vi "Config ACTION.vi"(8 "error in (no error)":errorcluster, 11 "Measurement in":refnum<class "Measurement.lvclass">) -> (0 "error out":errorcluster, 3 "Measurement out":refnum<class "Measurement.lvclass">)   [LabVIEW 2014, in "SeqLoop.lvlib" / "STEP Classes.lvlib" / "Measurement.lvclass"]
uses:
  Measurement.lvclass
  Resources/XControls/Selectable ListBox xControl/ListBox XControl.xctl
  Measurement.lvclass/Measurement.ctl
panel:
  in  "HWAsync Actions":T1={"HWAsync 1"="---", "HWAsync 2"="---", "HWAsync 3"="---", "HWAsync 4"="---", "HWAsync 5"="---", "HWAsync 6"="---", "HWAsync 7"="---", "HWAsync 8"="---", "HWAsync 9"="---", "HWAsync 10"="---"}
  in  "Deselect All":bool
  in  "Select All":bool
  in  "Cancel":bool
  in  "Save":bool
  in  "Measurement List":string[](xcontrol)
  # "Seleccione Mediciones a Calcular"
  # "Hardware Asíncronos"
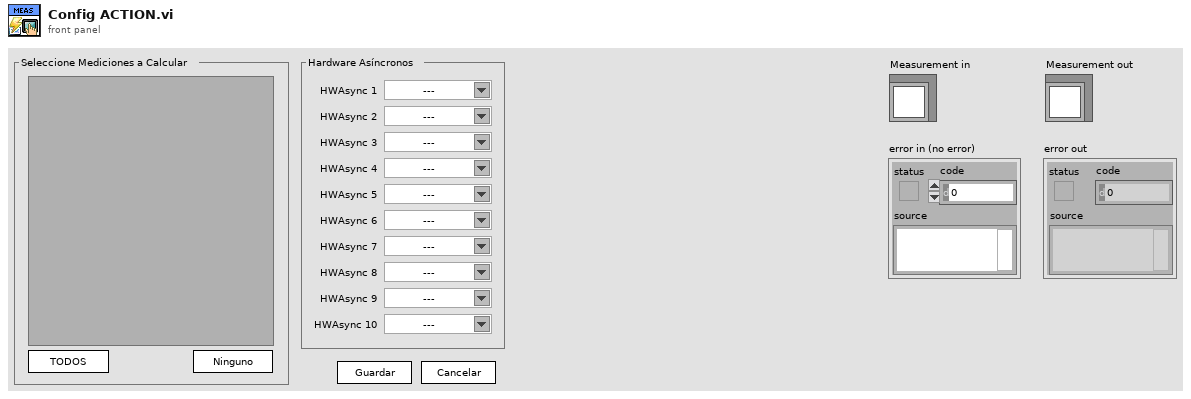
[diagram p1: front panel]
types:
  T1 = cluster{"HWAsync 1":string, "HWAsync 2":string, "HWAsync 3":string, "HWAsync 4":string, "HWAsync 5":string, "HWAsync 6":string, "HWAsync 7":string, "HWAsync 8":string, "HWAsync 9":string, "HWAsync 10":string}
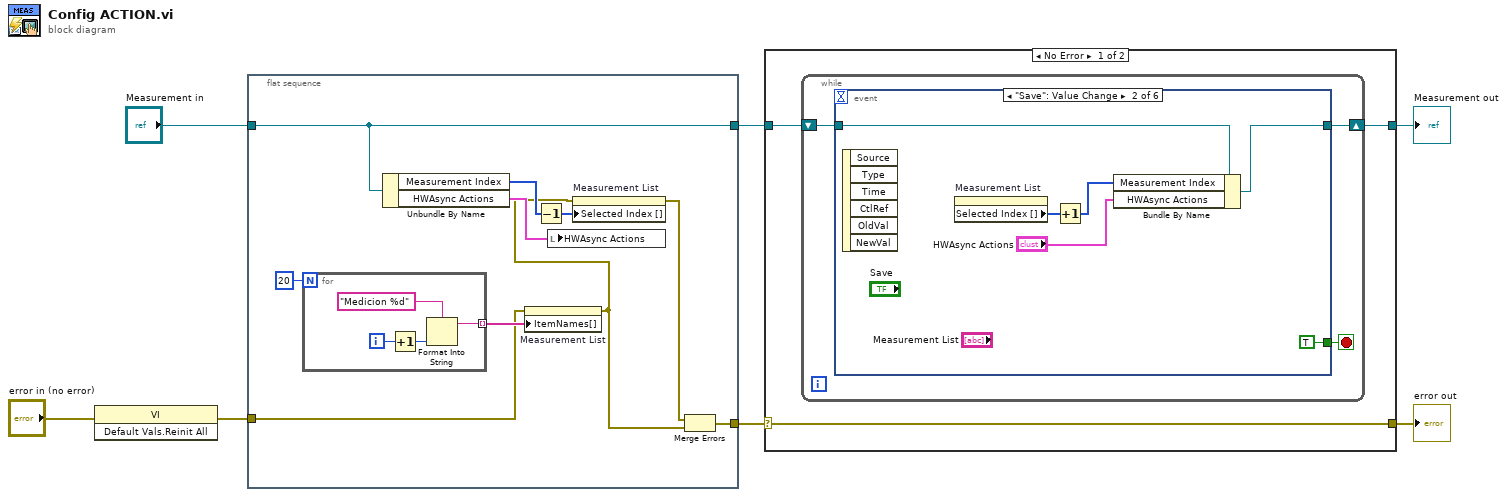
[diagram p0: block diagram]
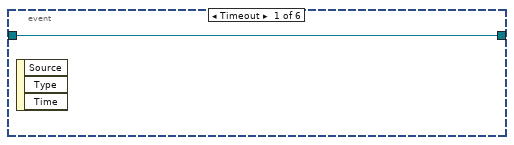
[diagram p2: hidden frame]
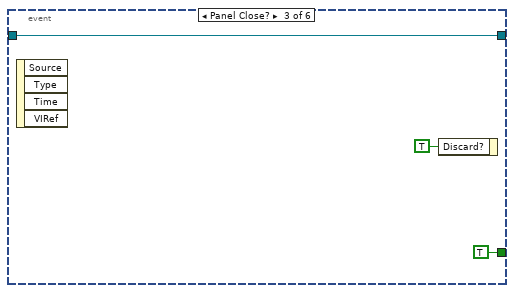
[diagram p3: hidden frame]
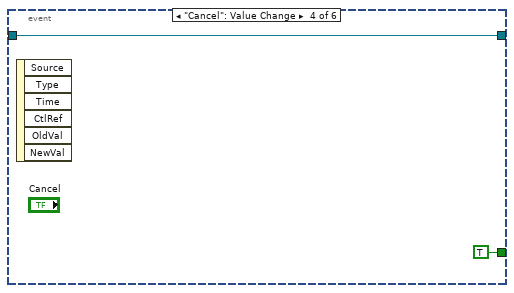
[diagram p4: hidden frame]
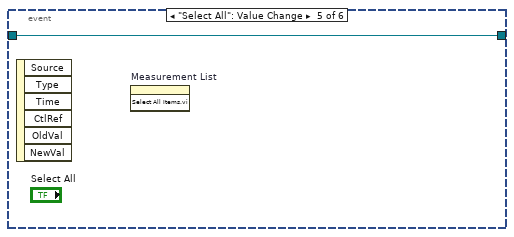
[diagram p5: hidden frame]
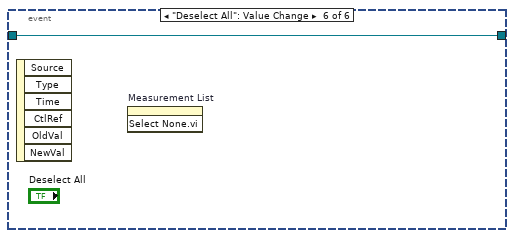
[diagram p6: hidden frame]
diagram:
  n1 = invoke class="VI" method="Default Vals.Reinit All"(error in="error in (no error)") -> (error out=w2:errorcluster)  [unwired: 2 in, 2 out]
  n2 = flat-sequence {
    tunnel: "Measurement in" -> [w10]
    tunnel: [w14] -> w4
    tunnel: w2 -> [w9]
    tunnel: [w10] -> w1
    frame #0 {
      n3 = for {
        N: 20 -> [_]
        tunnel: [w18] -> w17 mode=indexing
        i -> [w19]
        n4 = Increment(x=w19) -> (x+1=w20:i32)
        n5 = Format Into String(format string="Medicion %d", w20) -> (resulting string=w18:string)  [unwired: 2 in, 1 out]
      }
      n6 = Unbundle By Name(w10) -> ("Measurement Index"=w11:i32[], "HWAsync Actions"=w15:T1)
      n7 = property on="Measurement List" class="ListBox XControl (strict)"(error in=w9, "ItemNames[]"=w17) -> (error out=w8:errorcluster)  [unwired: 1 in, 1 out]
      n8 = Decrement(x=w11) -> (x-1=w12:i32[])
      n9 = local write "HWAsync Actions"(w15) -> ()
      n10 = property on="Measurement List" class="ListBox XControl (strict)"(error in=w8, "Selected Index []"=w12) -> (error out=w13:errorcluster)  [unwired: 1 in, 1 out]
      n11 = Merge Errors(w13, w8) -> (w14:errorcluster)
    }
  }
  n12 = case shown="No Error" w4 {
    selector: w4 -> [w24 w43]
    tunnel: [w24 w43] -> w7
    tunnel: [w22 w42] -> w6
    tunnel: w1 -> [w23 w42]
    frame No Error {
      n13 = while {
        shift-right: [w26] -> w22
        shift-left: w23 -> [w27]
        stop <- w25 stop-if-true
        n14 = event shown="[1] \"Save\": Value Change" {
          selector: _ -> [_ _ _ _ _ _]
          dyn-events: _ -> [_ _ _ _ _ _]
          timeout: _ -> [_ _ _ _ _ _]
          tunnel: w27 -> [w28 w32 w37 w39 w40 w41]
          tunnel: [w28 w31 w37 w39 w40 w41] -> w26
          tunnel: [_ TRUE TRUE TRUE _ _] -> w25
          event Timeout {
            n15 = event-data() -> ()  [unwired: 1 in, 3 out]
          }
          event "Save": Value Change {
            n16 = event-data() -> ()  [unwired: 1 in, 6 out]
            n17 = property on="Measurement List" class="ListBox XControl (strict)"() -> ("Selected Index []"=w30:i32[])  [unwired: 2 in, 2 out]
            n18 = Increment(x=w30) -> (x+1=w29:i32[])
            n19 = Bundle By Name(cluster=w32, "Measurement Index"=w29, "HWAsync Actions"="HWAsync Actions") -> (w31:refnum<class "Measurement.lvclass">)
          }
          event Panel Close? {
            n20 = event-data() -> ()  [unwired: 1 in, 4 out]
            n21 = event-data("Discard?"=TRUE) -> ()  [unwired: 1 in, 1 out]
          }
          event "Cancel": Value Change {
            n22 = event-data() -> ()  [unwired: 1 in, 6 out]
          }
          event "Select All": Value Change {
            n23 = event-data() -> ()  [unwired: 1 in, 6 out]
            n24 = invoke on="Measurement List" class="ListBox XControl (strict)" method="Select All Items.vi"() -> ()  [unwired: 3 in, 3 out]
          }
          event "Deselect All": Value Change {
            n25 = event-data() -> ()  [unwired: 1 in, 6 out]
            n26 = invoke on="Measurement List" class="ListBox XControl (strict)" method="Select None.vi"() -> ()  [unwired: 3 in, 3 out]
          }
        }
      }
    }
    frame Error {
    }
  }
  "error out" <- w7
  "Measurement out" <- w6
